vi "dfd_Super Narrowband Filter Design Masking Filter Design.vi"(5 "masking order":i32, 6 "CIC order":i32, 7 "filter type":T1(ring), 8 "error in (no error)":errorcluster, 10 "Masking band parameters":T7[](array[typedef])=[{"band specification"=[{"freq"=0.0, "amplitude"=1.0, "weight"=1.0}, {"freq"=0.2, "amplitude"=1.0, "weight"=1.0}], "ripple constraint"=0.0}, {"band specification"=[{"freq"=0.3, "amplitude"=0.0, "weight"=1.0}, {"freq"=0.5, "amplitude"=0.0, "weight"=1.0}], "ripple constraint"=0.0}], 11 "N":i32) -> (0 "error out":errorcluster, 3 "multirate filter out":T2={"mMRate_Structure"=enum."CIC", "mMRate_Mode"=0, "mMRate_Factor"=1, "mMRate_FIRParams"={"mMRate_FIR_H"=[], "mMRate_FIR_IsNyquist?"=FALSE, "mMRate_FIR_IsSymmetric?"=FALSE}, "mMRate_CICParams"={"mMRate_CIC_#Stage"=2, "mMRate_CIC_Lag"=1, "mMRate_CIC_Type"=enum."Lowpass"}, "mMRate_Order"=1, "mMRate_Version"="1.0", "mMRate_Comments"="1.0", "mMRate_RationalFactor"={"mMRate_L"=-1, "mMRate_M"=-1}, "mMRate_Fs"=1.0, "mMRate_Quantized?"=FALSE, "mMRate_QFilterGain"=1.0, "mMRate_CoefWl"=16, "mMRate_Scaling"={"mMRate_ScaleByPowerOf2?"=FALSE, "mMRate_ScaleType"=enum."Time Domain 1-Norm"}, "mMRate_InputWl"=0, "mMRate_OutputWl"=0, "mMRate_OutputMode"=enum."Nearest", "mMRate_MultMode"=enum."Truncated", "mMRate_BitPruning"=FALSE, "mMRate_GainWl"=16, "mMRate_OutputFwl"=0, "mMRate_SumIwl"=0, "mMRate_InputIwl "=16, "mMRate_SumWl"=32, "mMRate_CoefIwl"=0} {"mMRate_SumWl" min=1 max=32 step=1; "mMRate_InputIwl" min=1 max=32 step=1; "mMRate_GainWl" min=1 max=32 step=1; "mMRate_OutputWl" min=1 max=32 step=1; "mMRate_InputWl" min=1 max=32 step=1; "mMRate_CoefWl" min=1 max=32 step=1; "mMRate_Mode" items=["Default"=-1, "No Rate Change"=0, "Interpolation"=1, "Decimation"=2, "Interpolated"=3, "Rational"=4]})   [LabVIEW 2017, in "NI_DigFilter_Process.lvlib"]
uses:
  <vilib>/addons/Digital Filter Design/NI_DigFilter_Process.lvlib
  <vilib>/addons/Digital Filter Design/_Objects.llb/DFD Adv Band Spec.ctl
  <vilib>/addons/Digital Filter Design/_Objects.llb/DFD Multirate Filter Obj.ctl
  <vilib>/addons/Digital Filter Design/_Objects.llb/DFD Multirate Mode.ctl
  <vilib>/addons/Digital Filter Design/_Objects.llb/DFD Coef Norm Type.ctl
  <vilib>/addons/Digital Filter Design/_Objects.llb/DFD Round-off Mode.ctl
  <vilib>/addons/Digital Filter Design/_Objects.llb/DFD FXP MRate Multiply Mode.ctl
  <vilib>/addons/Digital Filter Design/_REMEZ.llb/remez_fir filter type.ctl
  <vilib>/addons/Digital Filter Design/NI_DigFilterLicensed.lvlib
panel:
  # "freq"
  # "amplitude"
  # "weight"
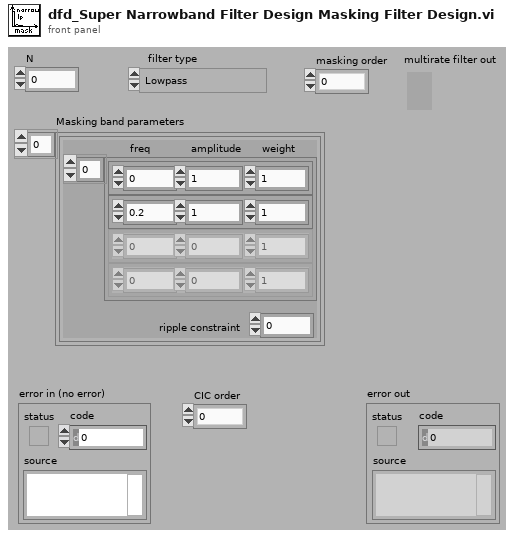
[diagram p1: front panel]
types:
  T1 = enum32{"Lowpass", "Highpass", "Bandpass", "Bandstop", "Wideband-Lowpass", "Wideband-Highpass"}
  T2 = typedef "NI_DigFilterLicensed.lvlib/DFD Multirate Filter Obj.ctl" = cluster{"mMRate_Structure":enum16{"CIC", "FIR", "IIR", "Lattice"}, "mMRate_Mode":T3, "mMRate_Factor":i32, "mMRate_FIRParams":cluster{"mMRate_FIR_H":dbl[], "mMRate_FIR_IsNyquist?":bool, "mMRate_FIR_IsSymmetric?":bool}, "mMRate_CICParams":cluster{"mMRate_CIC_#Stage":i32, "mMRate_CIC_Lag":i32, "mMRate_CIC_Type":enum16{"Lowpass", "Highpass"}}, "mMRate_Order":i32, "mMRate_Version":string, "mMRate_Comments":string, "mMRate_RationalFactor":cluster{"mMRate_L":i32, "mMRate_M":i32}, "mMRate_Fs":dbl, "mMRate_Quantized?":bool, "mMRate_QFilterGain":dbl, "mMRate_CoefWl":i16, "mMRate_Scaling":cluster{"mMRate_ScaleByPowerOf2?":bool, "mMRate_ScaleType":T4}, "mMRate_InputWl":i16, "mMRate_OutputWl":i16, "mMRate_OutputMode":T5, "mMRate_MultMode":T6, "mMRate_BitPruning":bool, "mMRate_GainWl":i16, "mMRate_OutputFwl":i16, "mMRate_SumIwl":i16, "mMRate_InputIwl ":i16, "mMRate_SumWl":i16, "mMRate_CoefIwl":i16}
  T3 = typedef "NI_DigFilterLicensed.lvlib/DFD Multirate Mode.ctl" = i16
  T4 = typedef "NI_DigFilterLicensed.lvlib/DFD Coef Norm Type.ctl" = enum16{"No Norm", "Time Domain 1-Norm", "Time Domain 2-Norm", "Time Domain Inf-Norm"}
  T5 = typedef "NI_DigFilterLicensed.lvlib/DFD Round-off Mode.ctl" = enum16{"Nearest", "Truncation"}
  T6 = typedef "NI_DigFilterLicensed.lvlib/DFD FXP MRate Multiply Mode.ctl" = enum16{"Truncated", "Full"}
  T7 = typedef "NI_DigFilterLicensed.lvlib/DFD Adv Band Spec.ctl" = cluster{"band specification":cluster{"freq":dbl, "amplitude":dbl, "weight":dbl}[], "ripple constraint":dbl}
  T8 = typedef "NI_DigFilterLicensed.lvlib/remez_fir filter type.ctl" = enum32{"Symmetric", "Antisymmetric", "Differentiator", "Hilbert", "Minimum Phase", "Maximum Phase"}
  T9 = typedef "NI_DigFilterLicensed.lvlib/DFD Filter Obj.ctl" = cluster{"mSRate_Fs":dbl, "mSRate_Version":string, "mSRate_Comments":string, "mSRate_OrgCoef":T10, "mSRate_CurCoef":T10, "mSRate_Quantized?":bool, "mSRate_QCoef":T10, "mSRate_QSettings":T12[], "mSRate_Order":i32, "mSRate_Scaling":cluster{"mSRate_ScaleByPowerOf2?":bool, "mSRate_ScaleType":T4}}
  T10 = typedef "NI_DigFilterLicensed.lvlib/DFD Filter Coef.ctl" = cluster{"type":T11, "gain":dbl, "coef a (k)":dbl[], "coef b (v)":dbl[]}
  T11 = typedef "NI_DigFilterLicensed.lvlib/DFD Filter Structure Type Selector.ctl" = enum16{"Undefined", "FIR Direct Form", "FIR Direct Form Transposed", "FIR Symmetric", "FIR Antisymmetric", "IIR Direct Form I", "IIR Direct Form I Transposed", "IIR Direct Form II", "IIR Direct Form II Transposed", "IIR Cascaded Second Order Sections Form I", "IIR Cascaded Second Order Sections Form I Transposed", "IIR Cascaded Second Order Sections Form II", "IIR Cascaded Second Order Sections Form II Transposed", "Lattice Allpass (basic sections)", "Lattice Allpass (one multiplier sections)", "Lattice Allpass (normalized sections)", "Lattice AR (basic sections)", "Lattice AR (one multiplier sections)", "Lattice AR (normalized sections)", "Lattice MA (minimum phase)", "Lattice MA (maximum phase)", "Lattice ARMA (basic sections)", "Lattice ARMA (one multiplier sections)", "Lattice ARMA (normalized sections)"}
  T12 = typedef "NI_DigFilterLicensed.lvlib/dfd_Internal Quantization Settings.ctl" = cluster{"source":T13, "wl":i16, "iwl":i16, "overflow mode":enum16{"Saturation", "Wrap"}, "rounding mode":enum16{"Nearest", "Truncation"}, "signed?":bool}
  T13 = typedef "NI_DigFilterLicensed.lvlib/dfd_Internal Quantization Srcs.ctl" = u16
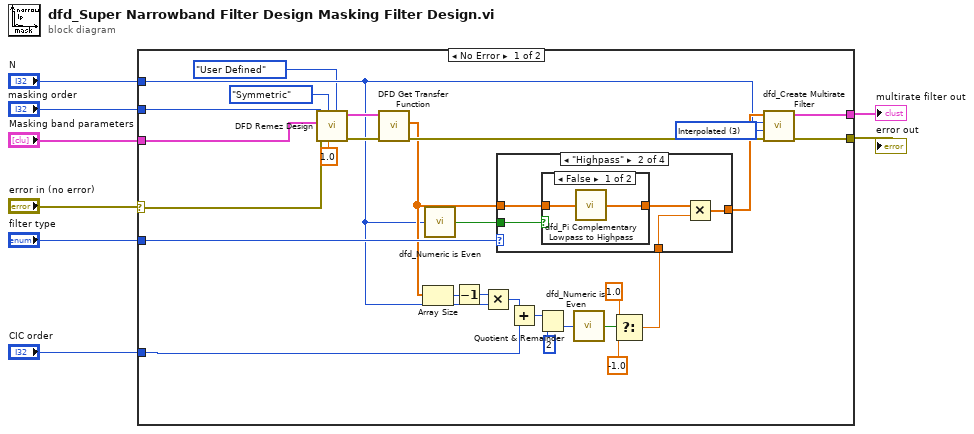
[diagram p0: block diagram]
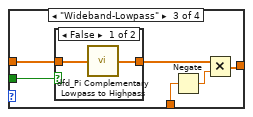
[diagram p4: hidden frame]
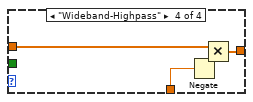
[diagram p6: hidden frame]
diagram:
  n1 = case shown="No Error" "error in (no error)" {
    selector: "error in (no error)" -> [w10 w59]
    tunnel: "N" -> [w16 _]
    tunnel: [w15 _] -> w7
    tunnel: [w14 w59] -> w6
    tunnel: "Masking band parameters" -> [w12 _]
    tunnel: "filter type" -> [w32 _]
    tunnel: "CIC order" -> [w20 _]
    tunnel: "masking order" -> [w11 _]
    frame No Error {
      w13 = T3 3 items=["Default"=-1, "No Rate Change"=0, "Interpolation"=1, "Decimation"=2, "Interpolated"=3] ("mode")
      n2 = call <vilib>:"DFD Remez Design.vi"("minimum order"=enum32{"User Defined", "MinEven", "MinOdd"}."User Defined", "fs [Hz]"=1.0 ("fs (Hz)"), "filter type"=remez_fir_filter_type."Symmetric", "error in (no error)"=w10, "band specs"=w12, "order"=w11) -> ("error out"=w35:errorcluster, "filter out"=w31:T9)  [unwired: 1 in, 3 out]
      n3 = call <vilib>:"DFD Get Transfer Function.vi"("error in (no error)"=w35, "filter in"=w31) -> ("error out"=w34:errorcluster, "numerator"=w30:dbl[])  [unwired: 8 out]
      n4 = Array Size(array=w30) -> (size(s)=w29:i32)
      n5 = call <vilib>:"dfd_Numeric is Even.vi"("N"=w16) -> ("even ?"=w33:bool)
      n6 = Decrement(x=w29) -> (x-1=w28:i32)
      n7 = Multiply(x=w28, y=w16) -> (x*y=w19:i32)
      n8 = Add(x=w19, y=w20) -> (x+y=w27:i32)
      n9 = Quotient & Remainder(x=w27, y=2) -> (floor(x/y)=w25:i32)  [unwired: 1 out]
      n10 = call <vilib>:"dfd_Numeric is Even.vi"("N"=w25) -> ("even ?"=w24:bool)
      n11 = Select(t=1.0, s=w24, f=-1.0) -> (s? t:f=w21:dbl)
      n12 = case shown="\"Highpass\"" w32 {
        tunnel: w30 -> [w37 w42 w51 w57]
        tunnel: [w37 w40 w49 w58] -> w17
        tunnel: w33 -> [_ w41 w50 _]
        tunnel: w21 -> [_ w38 w47 w56]
        frame "Lowpass", Default {
        }
        frame "Highpass" {
          n13 = case shown="False" w41 {
            tunnel: w42 -> [w44 w45]
            tunnel: [w43 w45] -> w39
            frame False {
              n14 = call <vilib>:"dfd_Pi Complementary Lowpass to Highpass.vi"("Lowpass"=w44) -> ("Highpass"=w43:dbl[])
            }
            frame True {
            }
          }
          n15 = Multiply(x=w39, y=w38) -> (x*y=w40:dbl[])
        }
        frame "Wideband-Lowpass" {
          n16 = case shown="False" w50 {
            tunnel: w51 -> [w53 w54]
            tunnel: [w52 w54] -> w48
            frame False {
              n17 = call <vilib>:"dfd_Pi Complementary Lowpass to Highpass.vi"("Lowpass"=w53) -> ("Highpass"=w52:dbl[])
            }
            frame True {
            }
          }
          n18 = Negate(x=w47) -> (-x=w46:dbl)
          n19 = Multiply(x=w48, y=w46) -> (x*y=w49:dbl[])
        }
        frame "Wideband-Highpass" {
          n20 = Negate(x=w56) -> (-x=w55:dbl)
          n21 = Multiply(x=w57, y=w55) -> (x*y=w58:dbl[])
        }
      }
      n22 = call <vilib>:"dfd_Create Multirate Filter.vi"("error in (no error)"=w34, "mode"=w13, "factor"=w16, "h (n)"=w17) -> ("error out"=w14:errorcluster, "multirate filter out"=w15:T2)  [unwired: 1 in, 5 out]
    }
    frame Error {
    }
  }
  "multirate filter out" <- w7
  "error out" <- w6
